vi "Low Pass Filter.vi"(6 "order":i32=2, 8 "Error In":errorcluster, 9 "Time constant":dbl=1.0, 10 "Sample rate":dbl=1.0, 11 "Data":cdb[](array[numeric])) -> (0 "Error Out":errorcluster, 3 "Data out":cdb[](array[numeric]))   [LabVIEW 2015]
uses:
  <vilib>/Analysis/3filter.llb/Filter Passband Type.ctl
  <vilib>/Analysis/3filter.llb/Butterworth Filter (CDB).vi
  <vilib>/Analysis/NI_AALBase.lvlib
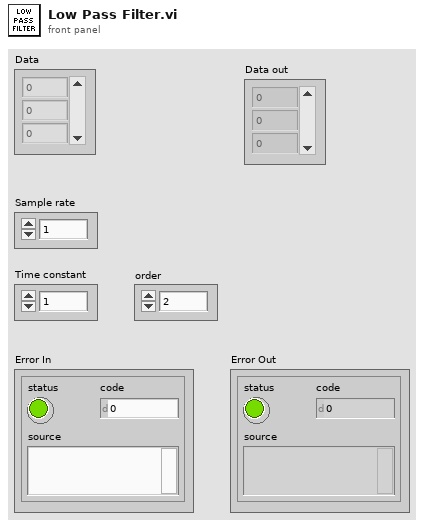
[diagram p1: front panel]
types:
  T1 = typedef "NI_AALBase.lvlib/Filter Passband Type.ctl" = enum32{"Lowpass", "Highpass", "Bandpass", "Bandstop"}
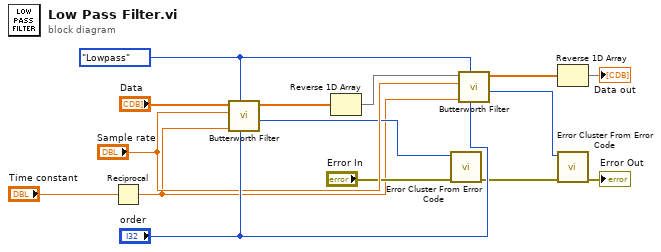
[diagram p0: block diagram]
diagram:
  w1 = Filter_Passband_Type."Lowpass" ("filter type")
  n1 = Reciprocal(x="Time constant") -> (1/x=w2:dbl)
  n2 = call-poly <vilib>:"Butterworth Filter.vi"("order"="order", "filter type"=w1, "low cutoff freq: fl"=w2, "sampling freq: fs"="Sample rate", "X"="Data") -> ("error"=w5:i32, "Filtered X"=w15:cdb[])  [unwired: 3 in]
  n3 = Reverse 1D Array(array=w15) -> (reversed array=w14:cdb[])
  n4 = call <vilib>:"Error Cluster From Error Code.vi"("error in (no error)"="Error In", "error code (0)"=w5) -> ("error out"=w8:errorcluster)  [unwired: 7 in]
  n5 = call-poly <vilib>:"Butterworth Filter.vi"("order"="order", "filter type"=w1, "low cutoff freq: fl"=w2, "sampling freq: fs"="Sample rate", "X"=w14) -> ("error"=w4:i32, "Filtered X"=w13:cdb[])  [unwired: 3 in]
  n6 = Reverse 1D Array(array=w13) -> (reversed array=→"Data out":cdb[])
  n7 = call <vilib>:"Error Cluster From Error Code.vi"("error in (no error)"=w8, "error code (0)"=w4) -> ("error out"=→"Error Out":errorcluster)  [unwired: 7 in]
